vi "Read Omni Bus.vi"(8 "error in (no error)":errorcluster, 11 "bt_WaitOn_Queue in":refnum<class "bt_WaitOn_Queue.lvclass">) -> (0 "error out":errorcluster, 2 "Omni_Bus.lvclass":refnum<class "Omni_Bus.lvclass">, 3 "bt_WaitOn_Queue out":refnum<class "bt_WaitOn_Queue.lvclass">)   [LabVIEW 2021, in "BT.lvlib" / "bt_WaitOn_Queue.lvclass"]
uses:
  bt_WaitOn_Queue.lvclass
  bt_WaitOn_Queue.lvclass/bt_WaitOn_Queue.ctl
  <vilib>/TSA/Omni-Bus/Omni-Bus/Omni_Bus.lvclass
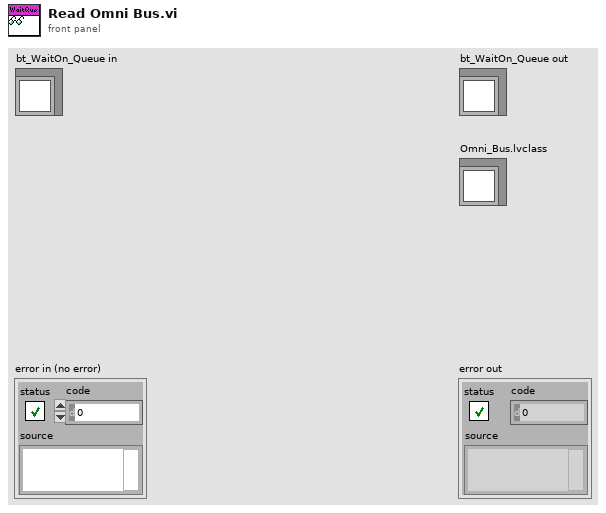
[diagram p1: front panel]
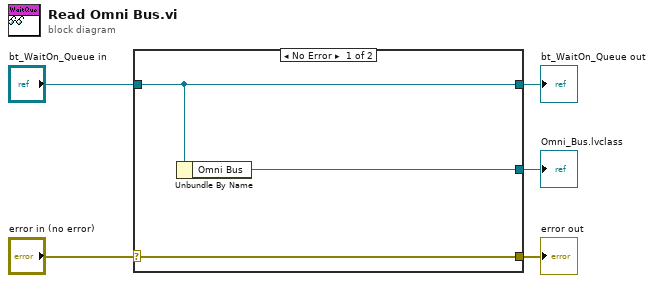
[diagram p0: block diagram]
diagram:
  n1 = case shown="No Error" "error in (no error)" {
    selector: "error in (no error)" -> [w8 w9]
    tunnel: [w8 w9] -> w4
    tunnel: [w7 w10] -> w2
    tunnel: "bt_WaitOn_Queue in" -> [w7 w10]
    tunnel: [w6 _] -> w1
    frame No Error {
      n2 = Unbundle By Name(w7) -> ("Omni Bus"=w6:refnum<class "Omni_Bus.lvclass">)
    }
    frame Error {
    }
  }
  "error out" <- w4
  "bt_WaitOn_Queue out" <- w2
  "Omni_Bus.lvclass" <- w1
